vi "Test Stop.vi"(11 "Error in":errorcluster) -> (15 "Error out":errorcluster)   [LabVIEW 2020, in "CelsiusToFarenheitTests.lvlib"]
doc: "This VI is to validate the stop button"
uses:
  CelsiusToFarenheitTests.lvlib
  <vilib>/SLL Drona/APIs/Assert/AssertVI/AssertVIExecRunning.vi
  <vilib>/SLL Drona/APIs/Stimulus/ControlValue/SetValueAuto.vi
  <vilib>/SLL Drona/APIs/Assert/AssertVI/AssertVIExecIdle.vi
  <vilib>/SLL Drona/APIs/Stimulus/VI/CloseVI.vi
  <vilib>/Utility/error.llb/Error Cluster From Error Code.vi
  <vilib>/ErrorRing/Error Ring.xnode
  <vilib>/SLL Drona/Drona.lvlib
  <vilib>/addons/_JKI Toolkits/Caraya/classes/Test/Test.lvclass
  <vilib>/Wiresmith Technology/G CLI/CLI Class/CLI.lvclass
  <vilib>/SLL Drona/APIs/Stimulus/VI/VI.lvlib
  <vilib>/SLL Drona/APIs/Assert/AssertVI/AssertVI.lvlib
  <vilib>/SLL Drona/APIs/Stimulus/ControlValue/ControlValue.lvlib
panel:
  # "STOP BUTTON TEST"
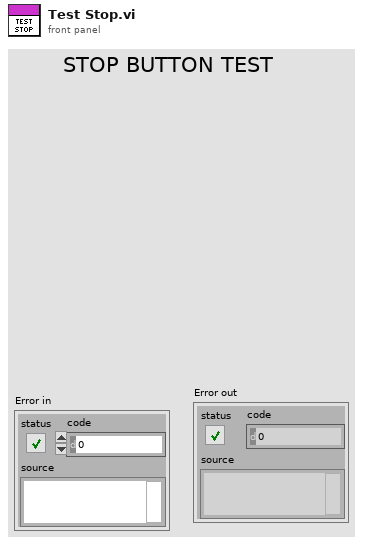
[diagram p1: front panel]
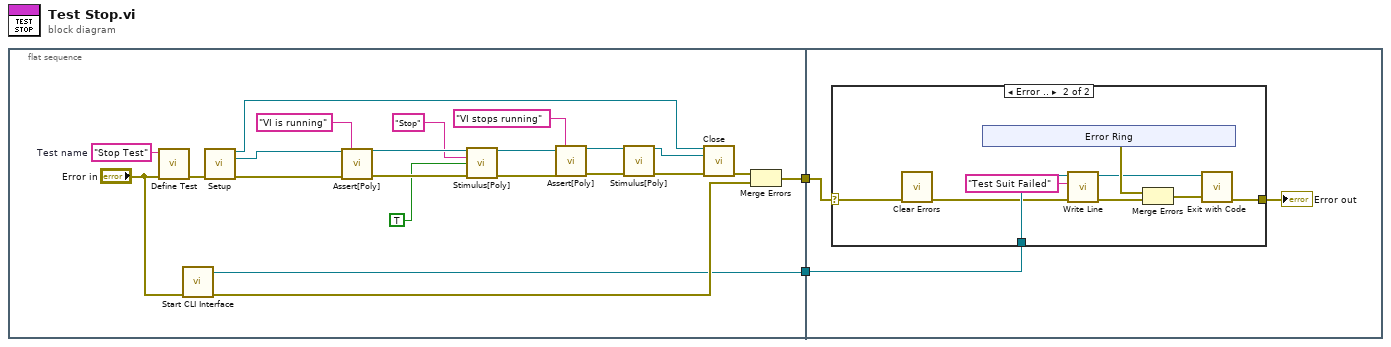
[diagram p0: block diagram]
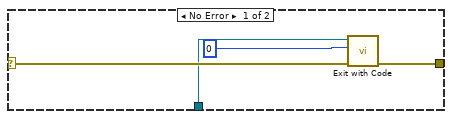
[diagram p2: hidden frame]
diagram:
  n1 = flat-sequence {
    tunnel: [w5] -> w2
    tunnel: [w3] -> w1
    tunnel: w2 -> [w27]
    tunnel: w1 -> [w25]
    frame #0 {
      w23 = "Stop Test"  # Test name
      n2 = call <vilib>:"Define Test.vi"("error in (no error)"="Error in", "Label (VI Title)"=w23) -> ("error out"=w24:errorcluster)  [unwired: 9 in]
      n3 = call <vilib>:"Start CLI Interface.vi"("error in (no error)"="Error in") -> ("error out"=w4:errorcluster, "CLI out"=w3:refnum<class "CLI.lvclass">)  [unwired: 7 in, 2 out]
      n4 = call <vilib>:"Setup.vi"("error in"=w24) -> ("Application Ref"=w22:refnum<vi>, "VI Reference Out"=w19:refnum<vi>, "error out"=w9:errorcluster)  [unwired: 12 in]
      n5 = call-poly <vilib>:"Assert[Poly].vi"("VI Reference In"=w19, "Test Label"="VI is running", "Error In"=w9) -> ("VI Reference Out"=w17:refnum<vi>, "Error Out"=w18:errorcluster)  [unwired: 11 in]
      n6 = call-poly <vilib>:"Stimulus[Poly].vi"("VI Reference In"=w17, "Control Path"="Stop", "Value (Signaling)"=TRUE, "error in"=w18) -> ("VI Reference Out"=w13:refnum<vi>, "error out"=w14:errorcluster)  [unwired: 10 in]
      n7 = call-poly <vilib>:"Assert[Poly].vi"("VI Reference In"=w13, "Test Label"="VI stops running", "Error In"=w14) -> ("VI Reference Out"=w10:refnum<vi>, "Error Out"=w11:errorcluster)  [unwired: 11 in]
      n8 = call-poly <vilib>:"Stimulus[Poly].vi"("VI Reference In"=w10, "error in"=w11) -> ("VI Reference Out"=w21:refnum<vi>, "error out"=w8:errorcluster)  [unwired: 12 in]
      n9 = call <vilib>:"Close.vi"("Application Ref"=w22, "VI Reference"=w21, "error in"=w8) -> ("error out"=w6:errorcluster)  [unwired: 12 in]
      n10 = Merge Errors(w6, w4) -> (w5:errorcluster)
    }
    frame #1 {
      n11 = case shown="Error .." w27 {
        selector: w27 -> [w29 w39]
        tunnel: [w31 w40] -> w26
        tunnel: w25 -> [w28 w38]
        frame No Error {
          n12 = call <vilib>:"Exit with Code.vi"("error in (no error)"=w29, "Exit Code (0)"=0, "CLI in"=w28) -> ("error out"=w31:errorcluster)  [unwired: 8 in]
        }
        frame Error {
          n13 = call <vilib>:"Clear Errors.vi"("error in (no error)"=w39) -> ("error out"=w32:errorcluster)  [unwired: 5 in, 1 out]
          n14 = xnode "Error Ring"() -> ("error out"=w35:errorcluster)
          n15 = call <vilib>:"Write Line.vi"("error in (no error)"=w32, "Text to Write"="Test Suit Failed", "CLI in"=w38) -> ("error out"=w34:errorcluster, "CLI out"=w33:refnum<class "CLI.lvclass">)  [unwired: 7 in]
          n16 = Merge Errors(w35, w34) -> (w36:errorcluster)
          n17 = call <vilib>:"Exit with Code.vi"("error in (no error)"=w36, "CLI in"=w33) -> ("error out"=w40:errorcluster)  [unwired: 9 in]
        }
      }
      "Error out" <- w26
    }
  }
